vi "LS_372_readout_still.vi"(4 "error in (no error)":errorcluster caption="Fehler (Eingang, kein Fehler)", 7 "VISA-Ressourcenname (in)":refnum<visa-resource-name>) -> (0 "error out":errorcluster caption="Fehler (Ausgang)", 2 "Still Value":dbl, 3 "VISA-Ressourcenname (out)":refnum<visa-resource-name>)   [LabVIEW 2019]
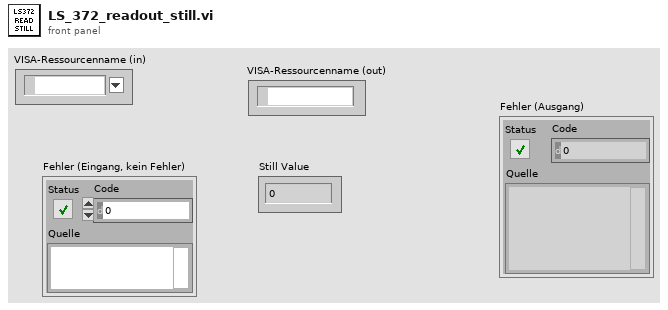
[diagram p1: front panel]
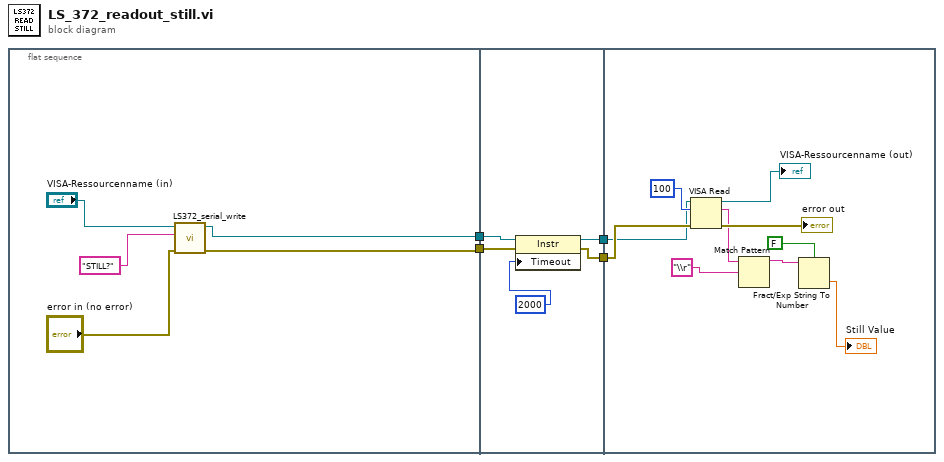
[diagram p0: block diagram]
diagram:
  n1 = flat-sequence {
    tunnel: [w8] -> w4
    tunnel: [w7] -> w3
    tunnel: w4 -> [w14]
    tunnel: w3 -> [w13]
    tunnel: [w11] -> w2
    tunnel: [w10] -> w1
    tunnel: w2 -> [w22]
    tunnel: w1 -> [w24]
    frame #0 {
      n2 = call "LS372_serial_write.vi"("error in (no error)"="error in (no error)", "Write Buffer (\"\")"="STILL?", "VISA resource name"="VISA-Ressourcenname (in)") -> ("error out"=w7:errorcluster, "VISA resource name out"=w8:refnum<visa-resource-name>)  [unwired: 6 in, 1 out]
    }
    frame #1 {
      n3 = property class="Instr"(reference=w14, error in=w13, "Timeout"=2000) -> (reference out=w11:refnum<visa-resource-name>, error out=w10:errorcluster)
    }
    frame #2 {
      n4 = VISA Read(VISA resource name=w22, byte count=100, error in (no error)=w24) -> (VISA resource name out=→"VISA-Ressourcenname (out)":refnum<visa-resource-name>, read buffer=w19:string, error out=→"error out":errorcluster)  [unwired: 1 out]
      n5 = Match Pattern(string=w19, regular expression="\\r") -> (before substring=w17:string)  [unwired: 1 in, 3 out]
      n6 = Fract/Exp String To Number(use system decimal point (T)=FALSE, string=w17) -> (number=→"Still Value":dbl)  [unwired: 2 in, 1 out]
    }
  }
